vi "SetSyncDeadTime.vi"(8 "error in (no error)":errorcluster, 9 "deadtime":i32, 10 "on":i32, 11 "Multiharp in":refnum<class "Multiharp.lvclass">) -> (0 "error out":errorcluster, 3 "Multiharp out":refnum<class "Multiharp.lvclass">)   [LabVIEW 2023, in "Multiharp.lvlib" / "Multiharp.lvclass"]
uses:
  Multiharp.lvclass
  <vilib>/ActorFramework/Actor/Actor.lvclass
  Multiharp Messages/InitHisto Msg/InitHisto Msg.lvclass
  MultiharpComm Messages/MH_ChannelInitDone Msg/MH_ChannelInitDone Msg.lvclass
  C:/Program Files/National Instruments/LabVIEW 2023/vi.lib/ActorFramework/Actor/Actor.lvclass
  C:/Users/quantum/Documents/LVDAQ/ConcreteClasses/ConcreteInstrumentClasses/Multiharp/Multiharp/Multiharp/Multiharp.lvclass
panel:
  in  "event data 2":cluster{"Init":bool, "nchannels":i32}
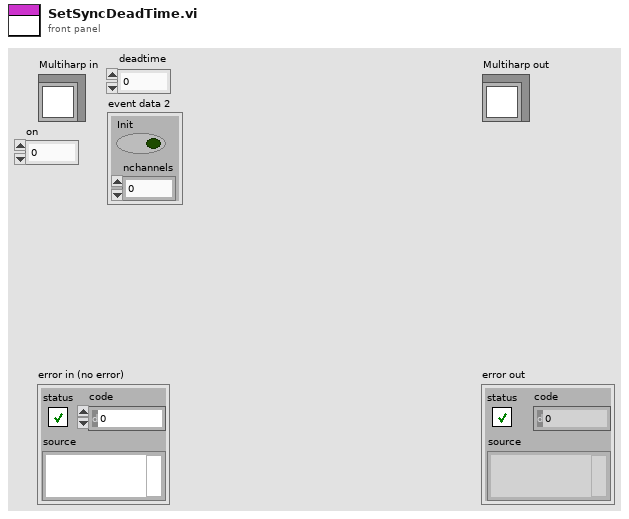
[diagram p1: front panel]
types:
  T1 = typedef "MH_MeasMode.ctl" = i32
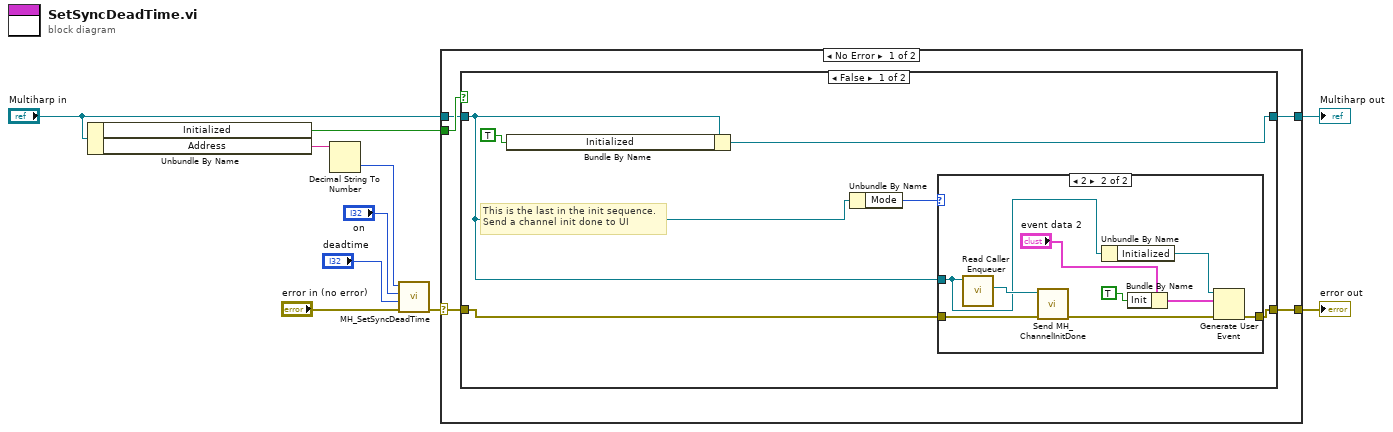
[diagram p0: block diagram]
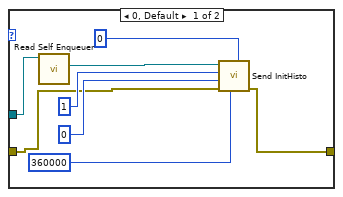
[diagram p2: hidden frame]
diagram:
  n1 = Unbundle By Name("Multiharp in") -> ("Initialized"=w7:bool, "Address"=w10:string)
  n2 = Decimal String To Number(string=w10) -> (number=w3:i32)  [unwired: 2 in, 1 out]
  n3 = call "MH_SetSyncDeadTime.vi"("error in (no error)"="error in (no error)", "deadtime"="deadtime", "on"="on", "devidx"=w3) -> ("error out"=w5:errorcluster)  [unwired: 6 in, 1 out]
  n4 = case shown="No Error" w5 {
    selector: w5 -> [w12 w41]
    tunnel: w7 -> [w15 _]
    tunnel: "Multiharp in" -> [w14 w42]
    tunnel: [w13 w42] -> w8
    tunnel: [w11 w41] -> w6
    frame No Error {
      n5 = case shown="False" w15 {
        tunnel: w14 -> [w17 w40]
        tunnel: [w20 w40] -> w13
        tunnel: w12 -> [w19 w39]
        tunnel: [w18 w39] -> w11
        frame False {
          # "This is the last in the init sequence.\nSend a channel init done to UI"
          n6 = Bundle By Name(cluster=w17, "Initialized"=TRUE ("InstrumentData.CurrentState.Initialized")) -> (w20:refnum<class "Multiharp.lvclass">)
          n7 = Unbundle By Name(w17) -> ("Mode"=w16:T1)
          n8 = case shown="2" w16 {
            tunnel: w19 -> [w25 w35]
            tunnel: [w24 w33] -> w18
            tunnel: w17 -> [w23 w30]
            frame 0, Default {
              n9 = call <vilib>:"Read Self Enqueuer.vi"("Actor"=w23) -> ("Self Enqueuer"=w29:refnum<class "Message Enqueuer.lvclass">)  [unwired: 10 in]
              n10 = call "Send InitHisto.vi"("lencode"=0, "tacq"=360000, "error in (no error)"=w25, "Offset"=0, "Binning"=1, "Message Enqueuer"=w29) -> ("error out"=w24:errorcluster)  [unwired: 4 in, 1 out]
            }
            frame 2 {
              n11 = call <vilib>:"Read Caller Enqueuer.vi"("Actor"=w30) -> ("Caller Enqueuer"=w31:refnum<class "Message Enqueuer.lvclass">)  [unwired: 10 in]
              n12 = call "Send MH_ChannelInitDone.vi"("error in (no error)"=w35, "Message Enqueuer"=w31) -> ("error out"=w38:errorcluster)  [unwired: 8 in, 1 out]
              n13 = Unbundle By Name(w30) -> ("Initialized"=w37:refnum<user-event>)
              n14 = Bundle By Name(cluster="event data 2", "Init"=TRUE) -> (w36:cluster{"Init":bool, "nchannels":i32})
              n15 = Generate User Event(user event=w37, event data cluster=w36, error in=w38) -> (error out=w33:errorcluster)  [unwired: 1 in, 1 out]
            }
          }
        }
        frame True {
        }
      }
    }
    frame Error {
    }
  }
  "error out" <- w6
  "Multiharp out" <- w8
